vi "ReceiveTCPfromPi_Binary.vi"() -> ()   [LabVIEW 2014]
uses:
  <vilib>/Utility/file.llb/Write To Spreadsheet File (string).vi
  <vilib>/Utility/file.llb/Write To Spreadsheet File (DBL).vi
panel:
  in  "Plot 3":u16(ring) items=["dT", "cT", "EKF VelN", "EKF VelE", "EKF VelD", "EKF PosN", "EKF PosE", "EKF PosD", "EKF Roll", "EKF Pitch", "EKF Yaw", "EKF Lat", "EKF Lon", "EKF Alt", "CMP VelN", "CMP VelE", "CMP VelD", "CMP PosN", "CMP PosE", "CMP PosD", "CMP Roll", "CMP Pitch", "CMP Yaw", "CMP Lat", "CMP Lon", "CMP Alt", "GPS Lat", "GPS Lon", "GPS Alt", "AccelX", "AccelY", "AccelZ", "GyroX", "GyroY", "GyroZ", "MagX", "MagY", "MagZ"]
  in  "Plot 2":u16(ring) items=["dT", "cT", "EKF VelN", "EKF VelE", "EKF VelD", "EKF PosN", "EKF PosE", "EKF PosD", "EKF Roll", "EKF Pitch", "EKF Yaw", "EKF Lat", "EKF Lon", "EKF Alt", "CMP VelN", "CMP VelE", "CMP VelD", "CMP PosN", "CMP PosE", "CMP PosD", "CMP Roll", "CMP Pitch", "CMP Yaw", "CMP Lat", "CMP Lon", "CMP Alt", "GPS Lat", "GPS Lon", "GPS Alt", "AccelX", "AccelY", "AccelZ", "GyroX", "GyroY", "GyroZ", "MagX", "MagY", "MagZ"]
  in  "Plot 1":u16(ring) items=["dT", "cT", "EKF VelN", "EKF VelE", "EKF VelD", "EKF PosN", "EKF PosE", "EKF PosD", "EKF Roll", "EKF Pitch", "EKF Yaw", "EKF Lat", "EKF Lon", "EKF Alt", "CMP VelN", "CMP VelE", "CMP VelD", "CMP PosN", "CMP PosE", "CMP PosD", "CMP Roll", "CMP Pitch", "CMP Yaw", "CMP Lat", "CMP Lon", "CMP Alt", "GPS Lat", "GPS Lon", "GPS Alt", "AccelX", "AccelY", "AccelZ", "GyroX", "GyroY", "GyroZ", "MagX", "MagY", "MagZ"]
  out "Num Characters Lost":i32
  in  "Spreadsheet Datalog File":path=path "C:/Users/romneyj/Desktop/EKFDatalog2.txt"
  in  "Binary Datalog File":path=path "C:/Users/romneyj/Desktop/EKFDatalog.txt"
  out "Chart Values":dbl[](array[numeric])
  out "Chart":cluster{"[0]":dbl, "[1]":dbl, "[2]":dbl}(graph)
  in  "Values to Display":dbl(slide)=100.0 min=10.0 max=2000.0 step=10.0 scale=10.0..2000.0
  out "error out":errorcluster
  out "before substring":string
  in  "stop":bool
  in  "Port":u16=5005
  in  "IP Address":string="155.31.242.65"
  # "Plot Values"
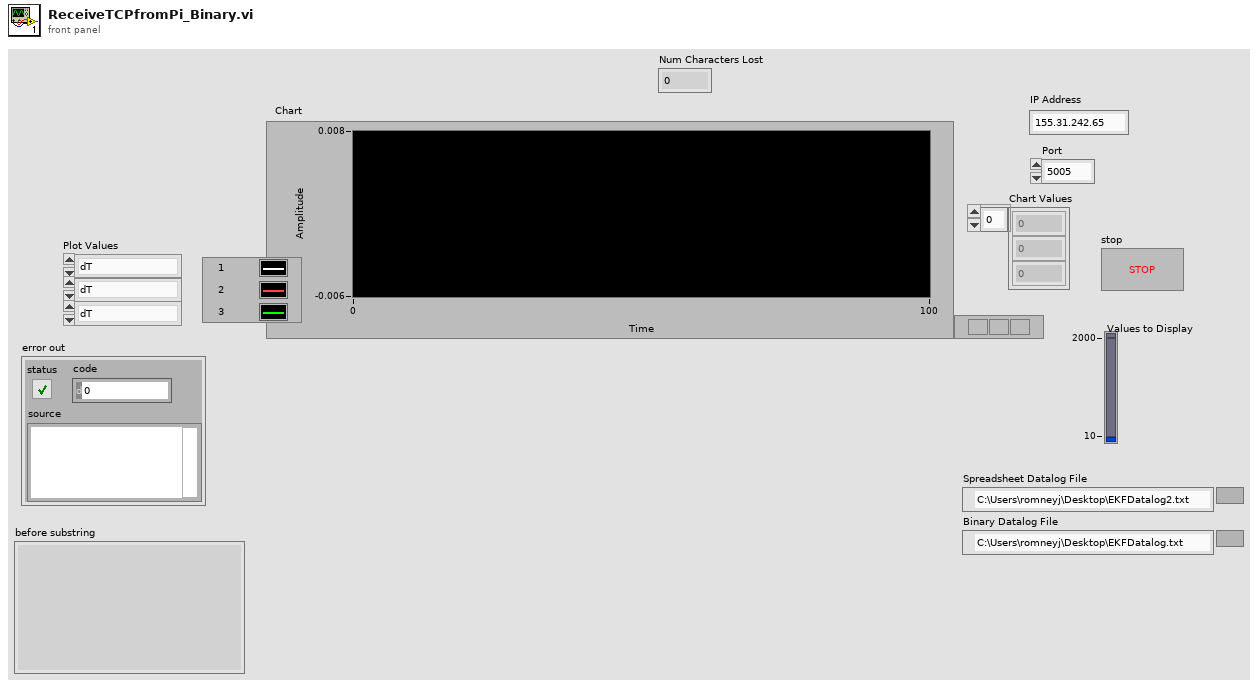
[diagram p1: front panel]
types:
  T1 = cluster{"dT":dbl, "cT":dbl, "EKF VelN":dbl, "EKF VelE":dbl, "EKF VelD":dbl, "EKF PosN":dbl, "EKF PosE":dbl, "EKF PosD":dbl, "EKF Roll":dbl, "EKF Pitch":dbl, "EKF Yaw":dbl, "EKF Lat":dbl, "EKF Lon":dbl, "EKF Alt":dbl, "CMP VelN":dbl, "CMP VelE":dbl, "CMP VelD":dbl, "CMP PosN":dbl, "CMP PosE":dbl, "CMP PosD":dbl, "CMP Roll":dbl, "CMP Pitch":dbl, "CMP Yaw":dbl, "CMP Lat":dbl, "CMP Lon":dbl, "CMP Alt":dbl, "GPS Lat":dbl, "GPS Lon":dbl, "GPS Alt":dbl, "AccelX":dbl, "AccelY":dbl, "AccelZ":dbl, "GyroX":dbl, "GyroY":dbl, "GyroZ":dbl, "MagX":dbl, "MagY":dbl, "MagZ":dbl}
  T2 = enum16{"open", "replace", "create", "open or create", "replace or create", "replace or create with confirmation"}
  T3 = enum16{"big-endian, network order", "native, host order", "little-endian"}
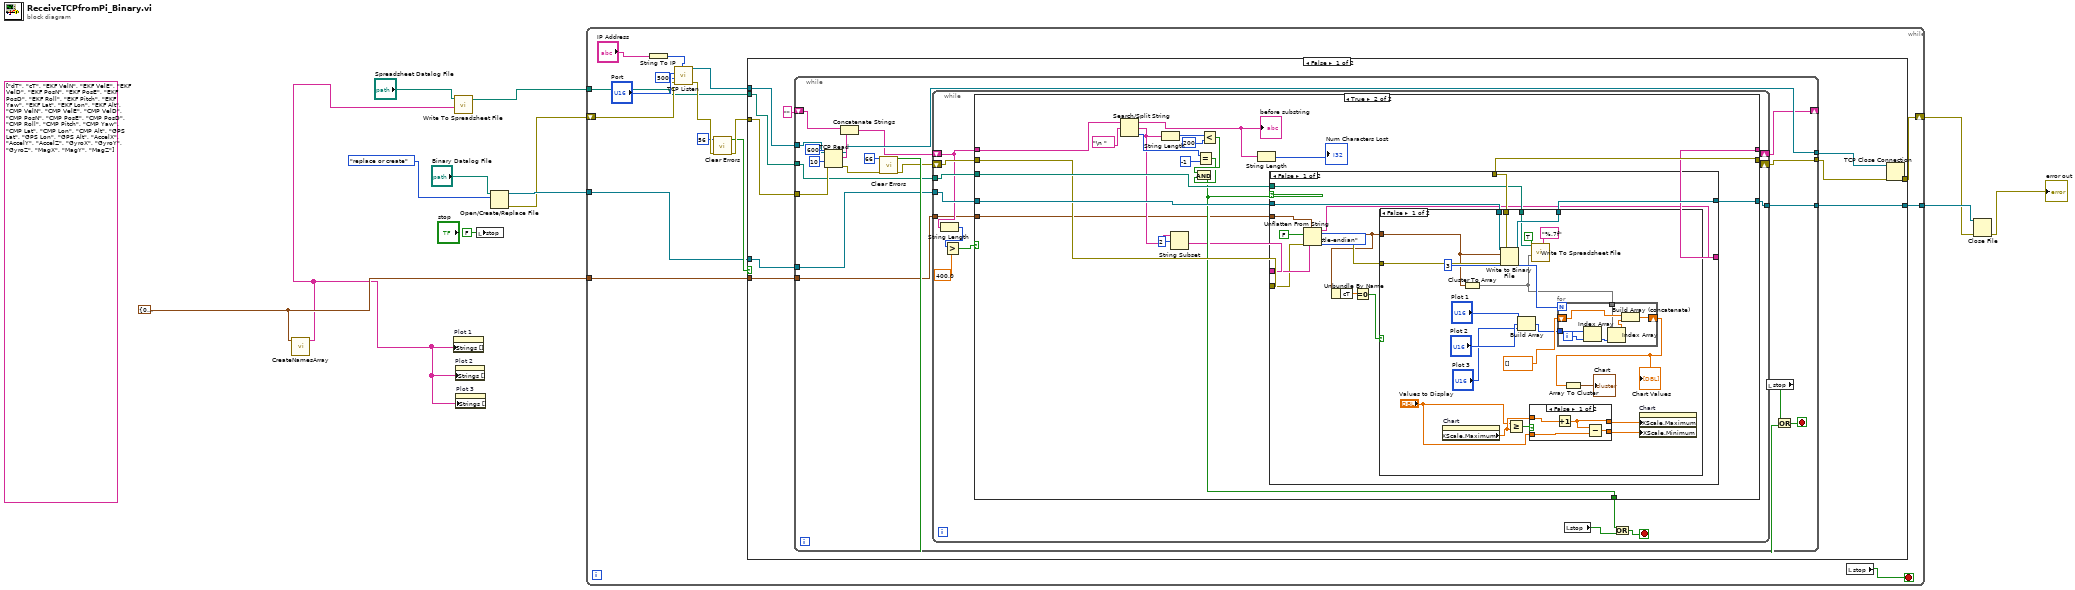
[diagram p0: block diagram]
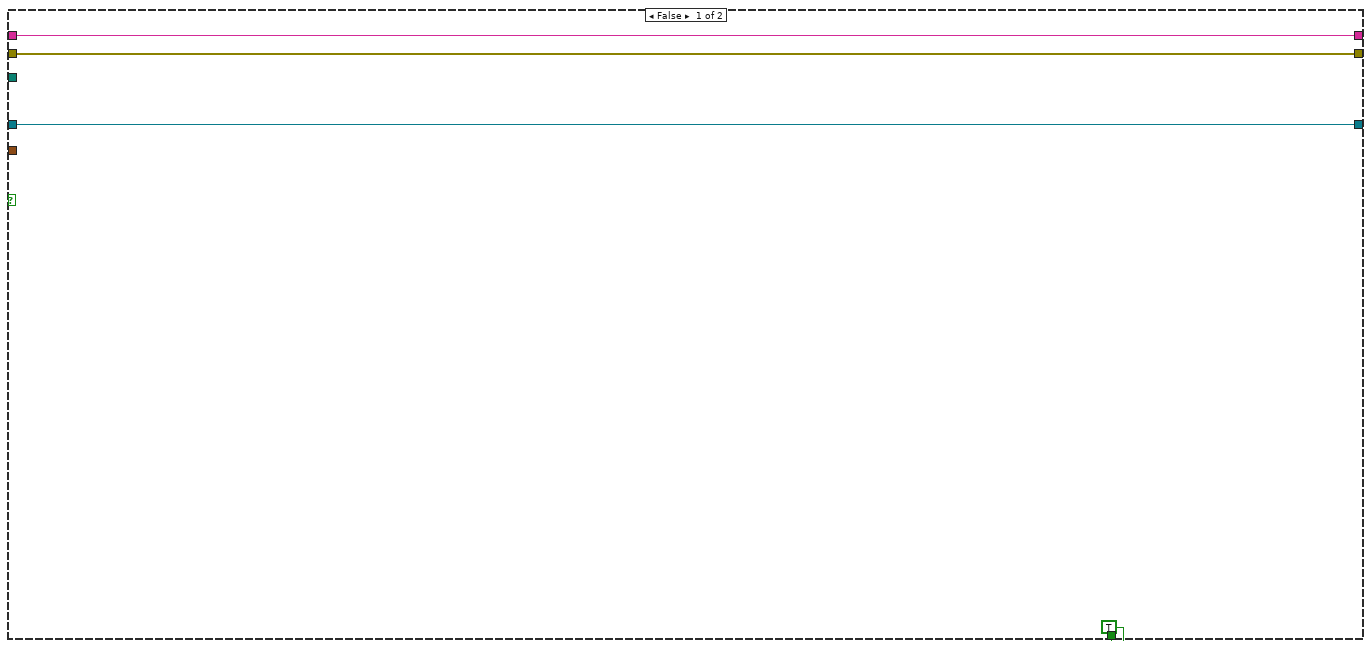
[diagram p2: hidden frame]
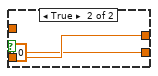
[diagram p3: hidden frame]
diagram:
  (unwired) string[] ["dT", "cT", "EKF VelN", "EKF VelE", "EKF VelD", "EKF PosN", "EKF PosE", "EKF PosD", "EKF Roll", "EKF Pitch", "EKF Yaw", "EKF Lat", "EKF Lon", "EKF Alt", "CMP VelN", "CMP VelE", "CMP VelD", "CMP PosN", "CMP PosE", "CMP PosD", "CMP Roll", "CMP Pitch", "CMP Yaw", "CMP Lat", "CMP Lon", "CMP Alt", "GPS Lat", "GPS Lon", "GPS Alt", "AccelX", "AccelY", "AccelZ", "GyroX", "GyroY", "GyroZ", "MagX", "MagY", "MagZ"] ("Array")
  w2 = T1 {"dT"=0.0, "cT"=0.0, "EKF VelN"=0.0, "EKF VelE"=0.0, "EKF VelD"=0.0, "EKF PosN"=0.0, "EKF PosE"=0.0, "EKF PosD"=0.0, "EKF Roll"=0.0, "EKF Pitch"=0.0, "EKF Yaw"=0.0, "EKF Lat"=0.0, "EKF Lon"=0.0, "EKF Alt"=0.0, "CMP VelN"=0.0, "CMP VelE"=0.0, "CMP VelD"=0.0, "CMP PosN"=0.0, "CMP PosE"=0.0, "CMP PosD"=0.0, "CMP Roll"=0.0, "CMP Pitch"=0.0, "CMP Yaw"=0.0, "CMP Lat"=0.0, "CMP Lon"=0.0, "CMP Alt"=0.0, "GPS Lat"=0.0, "GPS Lon"=0.0, "GPS Alt"=0.0, "AccelX"=0.0, "AccelY"=0.0, "AccelZ"=0.0, "GyroX"=0.0, "GyroY"=0.0, "GyroZ"=0.0, "MagX"=0.0, "MagY"=0.0, "MagZ"=0.0}
  n1 = call "CreateNamesArray.vi"("Cluster"=w2) -> ("Array"=w1:string[])  [unwired: 10 in]
  n2 = property on="Plot 1" class="Ring (strict)"("Strings []"=w1) -> ()  [unwired: 2 in, 2 out]
  n3 = call-poly <vilib>:"Write To Spreadsheet File.vi"("1D data"=w1, "file path (dialog if empty)"="Spreadsheet Datalog File") -> ("new file path (Not A Path if cancelled)"=w3:path)  [unwired: 6 in]
  n4 = property on="Plot 2" class="Ring (strict)"("Strings []"=w1) -> ()  [unwired: 2 in, 2 out]
  n5 = property on="Plot 3" class="Ring (strict)"("Strings []"=w1) -> ()  [unwired: 2 in, 2 out]
  n6 = local write "stop"(FALSE ("stop")) -> ()
  n7 = Open/Create/Replace File(file path (use dialog)="Binary Datalog File", operation (0:open)=T2."replace or create") -> (refnum out=w10:refnum<file>, error out=w5:errorcluster)  [unwired: 4 in, 1 out]
  n8 = while {
    shift-right: [w23] -> w8
    shift-left: w5 -> [w24]
    tunnel: w10 -> [w16]
    tunnel: [w15] -> w9
    tunnel: w3 -> [w14]
    tunnel: w2 -> [w13]
    stop <- w22 stop-if-true
    n9 = String To IP(1:"IP Address") -> (0:w26:u32)
    n10 = call <vilib>:"TCP Listen.vi"("net address"=w26, "error in (no error)"=w24, "timeout ms (wait forever: -1)"=500, "port"="Port") -> ("error out"=w20:errorcluster, "connection ID"=w25:refnum<k5>)  [unwired: 3 in, 3 out]
    n11 = call <vilib>:"Clear Errors.vi"("error in (no error)"=w20, "specific error code to clear (0: all)"=56) -> ("error out"=w19:errorcluster, "specific error cleared?"=w17:bool)  [unwired: 4 in]
    n12 = case shown="False" w17 {
      tunnel: w25 -> [w38 _]
      tunnel: [w34 w153] -> w23
      tunnel: w19 -> [w33 w153]
      tunnel: w16 -> [w32 w152]
      tunnel: [w31 w152] -> w15
      tunnel: w14 -> [w30 _]
      tunnel: w13 -> [w29 _]
      frame False {
        n13 = while {
          tunnel: w38 -> [w55]
          tunnel: w33 -> [w54]
          shift-right: [w50] -> _
          shift-left: "" -> [w53]
          tunnel: [w52] -> w36
          tunnel: [w51] -> w35
          tunnel: w32 -> [w42]
          tunnel: [w41] -> w31
          tunnel: w30 -> [w40]
          tunnel: w29 -> [w39]
          stop <- w45 stop-if-true
          n14 = TCP Read(connection ID=w55, bytes to read=600, error in (no error)=w54, 9:10 ("timeout ms (25000)")) -> (connection ID out=w52:refnum<k5>, data out=w58:string, error out=w44:errorcluster)  [unwired: 1 in]
          n15 = Concatenate Strings(w53, w58) -> (w49:string)
          n16 = call <vilib>:"Clear Errors.vi"("error in (no error)"=w44, "specific error code to clear (0: all)"=66 ("error code (no error:0)")) -> ("error out"=w43:errorcluster, "specific error cleared?"=w46:bool)  [unwired: 4 in]
          n17 = while {
            shift-right: [w71] -> w51
            shift-left: w43 -> [w72]
            shift-right: [w70] -> w50
            shift-left: w49 -> [w60]
            tunnel: w42 -> [w66]
            tunnel: [w65] -> w41
            tunnel: w40 -> [w64]
            tunnel: w39 -> [w59]
            stop <- w63 stop-if-true
            n18 = String Length(string=w60) -> (length=w68:i32)
            n19 = Greater?(x=w68, y=400.0) -> (0:w67:bool)
            n20 = case shown="True" w67 {
              tunnel: w72 -> [w75 w84]
              tunnel: w60 -> [w76 w92]
              tunnel: [w75 w95] -> w71
              tunnel: [w76 w85] -> w70
              tunnel: w66 -> [w74 w97]
              tunnel: [w74 w96] -> w65
              tunnel: w64 -> [_ w94]
              tunnel: [TRUE w83] -> w61
              tunnel: w59 -> [_ w77]
              frame False {
              }
              frame True {
                n21 = Search/Split String(string=w92, search string/char (-)="\n " ("regular expression")) -> (substring before match=w82:string, match + rest of string=w80:string, offset of match=w91:i32)  [unwired: 1 in]
                "before substring" <- w82
                n22 = String Length(string=w80) -> (length=w89:i32)
                n23 = String Subset(string=w80, offset (0)=2) -> (substring=w79:string)  [unwired: 1 in]
                n24 = Equal?(x=w91, y=-1) -> (x = y?=w86:bool)
                n25 = Less?(x=w89, y=200) -> (x < y?=w87:bool)
                n26 = And(x=w87, y=w86) -> (x .and. y?=w83:bool)
                n27 = String Length(string=w82) -> (length=→"Num Characters Lost":i32)
                n28 = case shown="False" w83 {
                  tunnel: w97 -> [w111 w151]
                  tunnel: [w110 w151] -> w96
                  tunnel: [w109 w150] -> w95
                  tunnel: w94 -> [w108 _]
                  tunnel: [w105 w149] -> w85
                  tunnel: w79 -> [w104 w149]
                  tunnel: w84 -> [w103 w150]
                  tunnel: w77 -> [w98 _]
                  frame False {
                    n29 = Unflatten From String(type=w98, binary string=w104, data includes array or string size? (T)=FALSE, byte order (0:big-endian, network order)=T3."little-endian", error in (no error)=w103) -> (rest of the binary string=w105:string, value=w101:T1, error out=w106:errorcluster)
                    n30 = Unbundle By Name(w101) -> ("cT"=w100:dbl)
                    n31 = Equal To 0?(x=w100) -> (x = 0?=w99:bool)
                    n32 = case shown="False" w99 {
                      tunnel: w111 -> [w133 w148]
                      tunnel: [w132 w148] -> w110
                      tunnel: [w131 w147] -> w109
                      tunnel: w108 -> [w128 _]
                      tunnel: w106 -> [w117 w147]
                      tunnel: w101 -> [w116 _]
                      frame False {
                        n33 = property on="Chart" class="WFChart (strict)"() -> ("XScale.Maximum"=w122:dbl)  [unwired: 2 in, 2 out]
                        n34 = Cluster To Array(cluster=w116) -> (array=w123:dbl[])
                        n35 = Write to Binary File(file (use dialog)=w133, data=w116, error in=w117) -> (refnum out=w132:refnum<file>, error out=w131:errorcluster)  [unwired: 3 in, 1 out]
                        n36 = Greater Or Equal?(x="Values to Display", y=w122) -> (x >= y?=w118:bool)
                        n37 = Build Array("Plot 1", "Plot 2", "Plot 3") -> (w115:u16[])
                        n38 = case shown="False" w118 {
                          tunnel: "Values to Display" -> [w136 w139]
                          tunnel: [w135 w139] -> w120
                          tunnel: [w137 0.0] -> w121
                          tunnel: w122 -> [w134 _]
                          frame False {
                            n39 = Increment(x=w134) -> (x+1=w135:dbl)
                            n40 = Subtract(x=w135, y=w136) -> (x-y=w137:dbl)
                          }
                          frame True {
                          }
                        }
                        n41 = call-poly <vilib>:"Write To Spreadsheet File.vi"("format (%.3f)"="%.7f", "append to file? (new file:F)"=TRUE, "1D data"=w123, "file path (dialog if empty)"=w128) -> ()  [unwired: 4 in, 1 out]
                        n42 = for {
                          N: 3 ("Number of Plots") -> [_]
                          tunnel: w115 -> [w145]
                          shift-right: [w140] -> w126
                          shift-left: dbl[] [] -> [w144]
                          tunnel: w123 -> [w142]
                          i -> [w143]
                          n43 = Index Array(array=w145, index=w143) -> (element=w146:u16)
                          n44 = Index Array(array=w142, index=w146) -> (element=w141:dbl)
                          n45 = Build Array (concatenate)(w144, w141) -> (w140:dbl[])
                        }
                        "Chart Values" <- w126
                        n46 = Array To Cluster(array=w126) -> (cluster=→"Chart":cluster{"[0]":dbl, "[1]":dbl, "[2]":dbl})
                        n47 = property on="Chart" class="WFChart (strict)"("XScale.Maximum"=w120, "XScale.Minimum"=w121) -> ()  [unwired: 2 in, 2 out]
                      }
                      frame True {
                      }
                    }
                  }
                  frame True {
                  }
                }
              }
            }
            n48 = local read "stop"() -> (w62:bool)
            n49 = Or(x=w61, y=w62) -> (x .or. y?=w63:bool)
          }
          n50 = local read "stop"() -> (w47:bool)
          n51 = Or(x=w47, y=w46) -> (x .or. y?=w45:bool)
        }
        n52 = TCP Close Connection(connection ID=w36, error in (no error)=w35) -> (error out=w34:errorcluster)  [unwired: 1 in, 1 out]
      }
      frame True {
      }
    }
    n53 = local read "stop"() -> (w22:bool)
  }
  n54 = Close File(refnum=w9, error in=w8) -> (error out=→"error out":errorcluster)  [unwired: 1 out]
